vi "log analysis_gps.vi"() -> ()   [LabVIEW 2018] (continued)
02000000,471d,15824;INS_ALIGNMENT_COMPLETE,INS_RTKFIXED,37.37068991155,126.72418127348,10.1440,22.3000,0.1660,-0.2361,-0.0346,-1.526557069,-2.043657004,301.319503447,0.4414,0.2936,0.5516,0.1147,0.0924,0.0773,0.0985,0.1037,4.8734,0f000001,0*5a4270f2\n\tsystem status\tnormal 2 28.000000 0 0\trobot status\t296.398114\t62.114495\t10.144000\t-1.526557\t-2.043657\t148.680497\t0.295000\t0.017000\n\t\n15:32:29.0\tlog_raw\tgps_raw\t\tsystem status\tnormal 2 28.000000 0 0\trobot status\t296.298636\t62.188359\t10.138000\t-1.401985\t-1.954148\t148.698075\t0.220000\t0.059000\n\t\n15:32:29.5\tlog_raw\tgps_raw\t\tsystem status\tnormal 2 28.000000 0 0\trobot status\t296.178072\t62.274593\t10.135400\t-1.361112\t-1.441905\t148.768068\t0.319000\t-0.040000\n\t\n15:32:30.0\tlog_raw\tgps_raw\t\tsystem status\tnormal 2 28.000000 0 0\trobot status\t296.075944\t62.352617\t10.130400\t-0.894382\t-1.568528\t148.753681\t0.263000\t0.005000\n\t\n15:32:30.5\tlog_raw\tgps_raw\t\tsystem status\tnormal 2 28.000000 0 0\trobot status\t295.964048\t62.434825\t10.132000\t-0.800917\t-1.256471\t148.752232\t0.304000\t-0.008000\n\t\n15:32:31.0\tlog_raw\tgps_raw\t\tsystem status\tnormal 2 28.000000 0 0\trobot status\t295.846178\t62.519865\t10.128900\t-0.939613\t-0.476224\t148.649480\t0.325000\t-0.046000\n\t\n15:32:31.5\tlog_raw\tgps_raw\t#INSPVAXA,USB3,0,52.5,FINESTEERING,2107,282769.500,02000000,471d,15824;INS_ALIGNMENT_COMPLETE,INS_RTKFIXED,37.37069431364,126.72417373673,10.1300,22.3000,0.1603,-0.2654,-0.0095,-1.268871738,-0.382060792,301.325978301,0.4464,0.2940,0.5510,0.1165,0.0927,0.0772,0.0984,0.1035,4.8643,0f000001,0*c8529f83\n\tsystem status\tnormal 2 28.000000 0 0\trobot status\t295.730521\t62.603083\t10.130000\t-1.268872\t-0.382061\t148.674022\t0.301000\t0.004000\n\t\n15:32:32.0\tlog_raw\tgps_raw\t\tsystem status\tnormal 2 28.000000 0 0\trobot status\t295.610868\t62.688092\t10.129000\t-1.384299\t-0.069981\t148.517098\t0.277000\t0.034000\n\t\n15:32:32.5\tlog_raw\tgps_raw\t\tsystem status\tnormal 2 28.000000 0 0\trobot status\t295.511357\t62.766081\t10.129700\t-1.066903\t0.012632\t148.592458\t0.294000\t-0.014000\n\t\n15:32:33.0\tlog_raw\tgps_raw\t\tsystem status\tnormal 2 28.000000 0 0\trobot status\t295.383113\t62.858245\t10.131300\t-1.221038\t-0.290292\t148.364562\t0.294000\t0.000000\n\t\n15:32:33.5\tlog_raw\tgps_raw\t#INSPVAXA,USB3,0,50.5,FINESTEERING,2107,282771.500,02000000,471d,15824;INS_ALIGNMENT_COMPLETE,INS_RTKFIXED,37.37069745960,126.72416836041,10.1313,22.3000,0.1734,-0.2561,-0.0200,-1.398091128,-0.585991174,301.767912429,0.4476,0.2943,0.5503,0.1154,0.0929,0.0772,0.0983,0.1033,4.8370,0f000001,0*46dd6173\n\tsystem status\tnormal 2 28.000000 0 0\trobot status\t295.254296\t62.952253\t10.131300\t-1.398091\t-0.585991\t148.232088\t0.306000\t0.007000\n\t\n15:32:34.0\tlog_raw\tgps_raw\t\tsystem status\tnormal 2 28.000000 0 0\trobot status\t295.144963\t63.032491\t10.131200\t-1.462857\t-0.836220\t148.096342\t0.289000\t-0.005000\n\t\n15:32:34.5\tlog_raw\tgps_raw\t\tsystem status\tnormal 2 28.000000 0 0\trobot status\t295.028200\t63.124039\t10.132500\t-1.207624\t-0.963061\t148.048115\t0.304000\t-0.003000\n\t\n15:32:35.0\tlog_raw\tgps_raw\t\tsystem status\tnormal 2 28.000000 0 0\trobot status\t294.908639\t63.216920\t10.132200\t-1.135657\t-1.024801\t147.963073\t0.305000\t0.001000\n\t\n15:32:35.5\tlog_raw\tgps_raw\t\tsystem status\tnormal 2 28.000000 0 0\trobot status\t294.793362\t63.307918\t10.132000\t-0.998560\t-1.105906\t147.899852\t0.305000\t0.003000\n\t\n15:32:36.0\tlog_raw\tgps_raw\t#INSPVAXA,USB3,0,48.0,FINESTEERING,2107,282774.000,02000000,471d,15824;INS_ALIGNMENT_COMPLETE,INS_RTKFIXED,37.37070158360,126.72416168804,10.1302,22.3000,0.1865,-0.2187,-0.0076,-0.878281232,-1.102464115,302.124757826,0.4458,0.2946,0.5497,0.1138,0.0924,0.0771,0.0982,0.1032,4.8072,0f000001,0*778beed4\n\tsystem status\tnormal 2 28.000000 0 0\trobot status\t294.663268\t63.409974\t10.130200\t-0.878281\t-1.102464\t147.875242\t0.297000\t0.008000\n\t\n15:32:36.5\tlog_raw\tgps_raw\t#INSPVAXA,USB3,0,51.0,FINESTEERING,2107,282774.500,02000000,471d,15824;INS_ALIGNMENT_COMPLETE,INS_RTKFIXED,37.37070240562,126.72416038344,10.1301,22.3000,0.1841,-0.2216,-0.0074,-0.755916604,-1.039971548,302.079440422,0.4445,0.2942,0.5497,0.1137,0.0923,0.0771,0.0982,0.1032,4.7994,0f000001,0*7d8abcba\n\tsystem status\tnormal 2 28.000000 0 0\trobot status\t294.547709\t63.501210\t10.130100\t-0.755917\t-1.039972\t147.920560\t0.257000\t0.069000\n\t\n15:32:37.0\tlog_raw\tgps_raw\t\tsystem status\tnormal 2 28.000000 0 0\trobot status\t294.441010\t63.584632\t10.130300\t-0.657644\t-1.098371\t147.886694\t0.256000\t0.071000\n\t\n15:32:37.5\tlog_raw\tgps_raw\t\tsystem status\tnormal 2 28.000000 0 0\trobot status\t294.326507\t63.674259\t10.129500\t-0.698609\t-0.924125\t147.966729\t0.306000\t0.009000\n\t\n15:32:38.0\tlog_raw\tgps_raw\t\tsystem status\tnormal 2 28.000000 0 0\trobot status\t294.207903\t63.767336\t10.127700\t-0.622193\t-0.914822\t148.095651\t0.389000\t-0.119000\n\t\n15:32:38.5\tlog_raw\tgps_raw\t\tsystem status\tnormal 2 28.000000 0 0\trobot status\t294.089085\t63.861289\t10.125200\t-0.528009\t-1.070164\t148.237491\t0.311000\t0.003000\n\t\n15:32:39.0\tlog_raw\tgps_raw\t#INSPVAXA,USB3,0,52.0,FINESTEERING,2107,282777.000,02000000,471d,15824;INS_ALIGNMENT_COMPLETE,INS_RTKFIXED,37.37070657070,126.72415376285,10.1217,22.3000,0.2035,-0.2369,-0.0150,-0.446978250,-1.366804369,301.502448560,0.4425,0.2939,0.5496,0.1135,0.0924,0.0771,0.0982,0.1032,4.7938,0f000001,0*25f2a73f\n\tsystem status\tnormal 2 27.900000 0 0\trobot status\t293.961268\t63.963490\t10.121700\t-0.446978\t-1.366804\t148.497551\t0.249000\t0.102000\n\t\n15:32:39.5\tlog_raw\tgps_raw\t#INSPVAXA,USB3,0,51.5,FINESTEERING,2107,282777.500,02000000,471d,15824;INS_ALIGNMENT_COMPLETE,INS_RTKFIXED,37.37070737696,126.72415245019,10.1203,22.3000,0.1993,-0.2523,-0.0201,-0.489054474,-1.485846051,301.354572444,0.4412,0.2937,0.5492,0.1134,0.0927,0.0771,0.0982,0.1032,4.7938,0f000001,0*c63e4195\n\tsystem status\tnormal 2 27.900000 0 0\trobot status\t293.844995\t64.052977\t10.120300\t-0.489054\t-1.485846\t148.645428\t0.261000\t0.068000\n\t\n15:32:40.0\tlog_raw\tgps_raw\t#INSPVAXA,USB3,0,51.5,FINESTEERING,2107,282778.000,02000000,471d,15824;INS_ALIGNMENT_COMPLETE,INS_RTKFIXED,37.37070818895,126.72415111526,10.1183,22.3000,0.1970,-0.2381,-0.0048,-0.588842364,-1.719100289,301.162178179,0.4412,0.2937,0.5492,0.1134,0.0927,0.0771,0.0982,0.1032,4.7938,0f000001,0*cff0a9c3\n\tsystem status\tnormal 2 27.900000 0 0\trobot status\t293.726749\t64.143099\t10.118300\t-0.588842\t-1.719100\t148.837822\t0.260000\t0.055000\n\t\n15:32:40.5\tlog_raw\tgps_raw\t\tsystem status\tnormal 2 27.900000 0 0\trobot status\t293.621224\t64.222231\t10.114600\t-0.699985\t-1.731559\t149.030117\t0.234000\t0.109000\n\t\n15:32:41.0\tlog_raw\tgps_raw\t\tsystem status\tnormal 2 27.900000 0 0\trobot status\t293.505904\t64.308514\t10.110100\t-0.736273\t-1.630904\t149.356604\t0.241000\t0.105000\n\t\n15:32:41.5\tlog_raw\tgps_raw\t\tsystem status\tnormal 2 27.900000 0 0\trobot status\t293.392001\t64.394601\t10.106100\t-0.697006\t-1.585321\t149.593266\t0.253000\t0.078000\n\t\n15:32:42.0\tlog_raw\tgps_raw\t#INSPVAXA,USB3,0,45.0,FINESTEERING,2107,282780.000,02000000,471d,15824;INS_ALIGNMENT_COMPLETE,INS_RTKFIXED,37.37071131338,126.72414591828,10.1018,22.3000,0.1785,-0.2324,-0.0069,-0.645891836,-1.424803808,300.174839081,0.4413,0.2936,0.5502,0.1138,0.0926,0.0771,0.0982,0.1032,4.7947,0f000001,0*1d8f369d\n\tsystem status\tnormal 2 27.900000 0 0\trobot status\t293.266409\t64.489879\t10.101800\t-0.645892\t-1.424804\t149.825161\t0.271000\t0.042000\n\t\n15:32:42.5\tlog_raw\tgps_raw\t#INSPVAXA,USB3,0,47.0,FINESTEERING,2107,282780.500,02000000,471d,15824;INS_ALIGNMENT_COMPLETE,INS_RTKFIXED,37.37071208302,126.72414463488,10.0975,22.3000,0.1821,-0.2419,-0.0019,-0.556153794,-1.244614265,299.928543824,0.4419,0.2936,0.5508,0.1139,0.0925,0.0772,0.0982,0.1033,4.7946,0f000001,0*8f6fb982\n\tsystem status\tnormal 2 27.900000 0 0\trobot status\t293.152727\t64.575301\t10.097500\t-0.556154\t-1.244614\t150.071456\t0.269000\t0.063000\n\t\n15:32:43.0\tlog_raw\tgps_raw\t\tsystem status\tnormal 2 27.900000 0 0\trobot status\t293.049344\t64.652245\t10.092300\t-0.644835\t-1.201618\t150.236627\t0.241000\t0.104000\n\t\n15:32:43.5\tlog_raw\tgps_raw\t\tsystem status\tnormal 2 27.900000 0 0\trobot status\t292.934873\t64.737506\t10.087900\t-0.697254\t-1.176763\t150.373079\t0.274000\t0.036000\n\t\n15:32:44.0\tlog_raw\tgps_raw\t\tsystem status\tnormal 2 28.000000 0 0\trobot status\t292.821781\t64.822770\t10.082600\t-0.786091\t-1.232027\t150.520228\t0.272000\t0.043000\n\t\n15:32:44.5\tlog_raw\tgps_raw\t\tsystem status\tnormal 2 28.000000 0 0\trobot status\t292.705956\t64.906619\t10.078200\t-0.895000\t-1.549317\t150.670841\t0.281000\t0.039000\n\t\n15:32:45.0\tlog_raw\tgps_raw\t\tsystem status\tnormal 2 28.000000 0 0\trobot status\t292.590094\t64.991528\t10.072700\t-1.014159\t-1.880712\t150.764788\t0.241000\t0.093000\n\t\n15:32:45.5\tlog_raw\tgps_raw\t#INSPVAXA,USB3,0,52.5,FINESTEERING,2107,282783.500,02000000,471d,15824;INS_ALIGNMENT_COMPLETE,INS_RTKFIXED,37.37071667102,126.72413686312,10.0669,22.3000,0.1872,-0.2243,-0.0265,-0.901347734,-1.882595886,299.189069382,0.4437,0.2938,0.5525,0.1145,0.0924,0.0772,0.0982,0.1033,4.7951,0f000001,0*f21a15f8\n\tsystem status\tnormal 2 27.900000 0 0\trobot status\t292.464317\t65.084523\t10.066900\t-0.901348\t-1.882596\t150.810931\t0.334000\t-0.050000\n\t\n15:32:46.0\tlog_raw\tgps_raw\t#INSPVAXA,USB3,0,52.5,FINESTEERING,2107,282784.000,02000000,471d,15824;INS_ALIGNMENT_COMPLETE,INS_RTKFIXED,37.37071744310,126.72413557177,10.0615,22.3000,0.1842,-0.2203,-0.0202,-0.879207865,-1.728416069,299.181717490,0.4437,0.2938,0.5525,0.1145,0.0924,0.0772,0.0982,0.1033,4.7951,0f000001,0*6c7250dc\n\tsystem status\tnormal 2 28.000000 0 0\trobot status\t292.349932\t65.170216\t10.061500\t-0.879208\t-1.728416\t150.818283\t0.349000\t-0.068000\n\t\n15:32:46.5\tlog_raw\tgps_raw\t\tsystem status\tnormal 2 28.000000 0 0\trobot status\t292.247312\t65.245763\t10.056700\t-0.854639\t-1.542951\t150.875128\t0.263000\t0.061000\n\t\n15:32:47.0\tlog_raw\tgps_raw\t\tsystem status\tnormal 2 28.000000 0 0\trobot status\t292.131081\t65.329733\t10.048500\t-1.142793\t-1.256443\t150.916580\t0.255000\t0.070000\n\t\n15:32:47.5\tlog_raw\tgps_raw\t\tsystem status\tnormal 2 28.000000 0 0\trobot status\t292.014685\t65.414370\t10.039300\t-1.007102\t-1.150012\t150.972707\t0.245000\t0.079000\n\t\n15:32:48.0\tlog_raw\tgps_raw\t#INSPVAXA,USB3,0,48.5,FINESTEERING,2107,282786.000,02000000,471d,15824;INS_ALIGNMENT_COMPLETE,INS_RTKFIXED,37.37072048781,126.72413033534,10.0312,22.3000,0.2068,-0.2374,-0.0322,-0.835692120,-1.272043539,298.989138355,0.4439,0.2941,0.5534,0.1141,0.0925,0.0773,0.0982,0.1033,4.7952,0f000001,0*6862fbb7\n\tsystem status\tnormal 2 28.000000 0 0\trobot status\t291.886097\t65.508148\t10.031200\t-0.835692\t-1.272044\t151.010862\t0.396000\t-0.131000\n\t\n15:32:48.5\tlog_raw\tgps_raw\t#INSPVAXA,USB3,0,50.0,FINESTEERING,2107,282786.500,02000000,471d,15824;INS_ALIGNMENT_COMPLETE,INS_RTKFIXED,37.37072125488,126.72412899591,10.0263,22.3000,0.1993,-0.2318,-0.0321,-0.677738340,-1.537504569,298.882185903,0.4440,0.2942,0.5536,0.1140,0.0923,0.0773,0.0982,0.1033,4.7960,0f000001,0*3cb3310e\n\tsystem status\tnormal 2 28.000000 0 0\trobot status\t291.767453\t65.593285\t10.026300\t-0.677738\t-1.537505\t151.117814\t0.286000\t0.021000\n\t\n15:32:49.0\tlog_raw\tgps_raw\t#INSPVAXA,USB3,0,50.0,FINESTEERING,2107,282787.000,02000000,471d,15824;INS_ALIGNMENT_COMPLETE,INS_RTKFIXED,37.37072202374,126.72412763229,10.0205,22.3000,0.2013,-0.2217,-0.0210,-0.794961813,-1.788062217,298.885711292,0.4440,0.2942,0.5536,0.1140,0.0923,0.0773,0.0982,0.1033,4.7960,0f000001,0*1f81862e\n\tsystem status\tnormal 2 28.000000 0 0\trobot status\t291.646666\t65.678621\t10.020500\t-0.794962\t-1.788062\t151.114289\t0.254000\t0.061000\n\t\n15:32:49.5\tlog_raw\tgps_raw\t#INSPVAXA,USB3,0,44.0,FINESTEERING,2107,282787.500,02000000,471d,15824;INS_ALIGNMENT_COMPLETE,INS_RTKFIXED,37.37072277220,126.72412626224,10.0147,22.3000,0.2002,-0.2137,-0.0290,-0.849980745,-1.812919554,298.887708696,0.4445,0.2943,0.5539,0.1141,0.0924,0.0773,0.0982,0.1034,4.7971,0f000001,0*c9e15001\n\tsystem status\tnormal 2 28.000000 0 0\trobot status\t291.525309\t65.761693\t10.014700\t-0.849981\t-1.812920\t151.112291\t0.307000\t-0.016000\n\t\n15:32:50.0\tlog_raw\tgps_raw\t#INSPVAXA,USB3,0,44.0,FINESTEERING,2107,282788.000,02000000,471d,15824;INS_ALIGNMENT_COMPLETE,INS_RTKFIXED,37.37072352565,126.72412491087,10.0076,22.3000,0.2060,-0.2242,-0.0325,-0.865126530,-1.802719391,298.872730955,0.4445,0.2943,0.5539,0.1141,0.0924,0.0773,0.0982,0.1034,4.7971,0f000001,0*c2266642\n\tsystem status\tnormal 2 28.000000 0 0\trobot status\t291.405607\t65.845318\t10.007600\t-0.865127\t-1.802719\t151.127269\t0.283000\t0.031000\n\t\n15:32:50.5\tlog_raw\tgps_raw\t#INSPVAXA,USB3,0,49.0,FINESTEERING,2107,282788.500,02000000,471d,15824;INS_ALIGNMENT_COMPLETE,INS_RTKFIXED,37.37072428040,126.72412354813,10.0007,22.3000,0.2098,-0.2286,-0.0305,-0.732817876,-1.872220332,298.881417220,0.4449,0.2943,0.5542,0.1142,0.0924,0.0773,0.0982,0.1034,4.7982,0f000001,0*a1e1a8aa\n\tsystem status\tnormal 2 28.000000 0 0\trobot status\t291.284897\t65.929088\t10.000700\t-0.732818\t-1.872220\t151.118583\t0.285000\t0.019000\n\t\n15:32:51.0\tlog_raw\tgps_raw\t#INSPVAXA,USB3,0,49.0,FINESTEERING,2107,282789.000,02000000,471d,15824;INS_ALIGNMENT_COMPLETE,INS_RTKFIXED,37.37072504347,126.72412218219,9.9929,22.3000,0.1951,-0.2277,-0.0250,-0.679984989,-2.019858796,298.956218881,0.4449,0.2943,0.5542,0.1142,0.0924,0.0773,0.0982,0.1034,4.7982,0f000001,0*d14e3525\n\tsystem status\tnormal 2 28.000000 0 0\trobot status\t291.163905\t66.013781\t9.992900\t-0.679985\t-2.019859\t151.043781\t0.288000\t0.011000\n\t\n15:32:51.5\tlog_raw\tgps_raw\t#INSPVAXA,USB3,0,50.5,FINESTEERING,2107,282789.500,02000000,471d,15824;INS_ALIGNMENT_COMPLETE,INS_RTKFIXED,37.37072577695,126.72412082127,9.9869,22.3000,0.2017,-0.2348,-0.0299,-0.707518535,-2.196709608,298.969096628,0.4457,0.2945,0.5546,0.1143,0.0924,0.0773,0.0982,0.1035,4.7994,0f000001,0*e2b500de\n\tsystem status\tnormal 2 28.000000 0 0\trobot status\t291.043357\t66.095190\t9.986900\t-0.707519\t-2.196710\t151.030903\t0.364000\t-0.092000\n\t\n15:32:52.0\tlog_raw\tgps_raw\t#INSPVAXA,USB3,0,50.5,FINESTEERING,2107,282790.000,02000000,471d,15824;INS_ALIGNMENT_COMPLETE,INS_RTKFIXED,37.37072651838,126.72411947234,9.9801,22.3000,0.2152,-0.2350,-0.0246,-0.689288795,-2.210478200,298.973213622,0.4457,0.2945,0.5546,0.1143,0.0924,0.0773,0.0982,0.1035,4.7994,0f000001,0*67dd8a4d\n\tsystem status\tnormal 2 28.000000 0 0\trobot status\t290.923871\t66.177482\t9.980100\t-0.689289\t-2.210478\t151.026786\t0.291000\t0.031000\n\t\n15:32:52.5\tlog_raw\tgps_raw\t#INSPVAXA,USB3,0,50.0,FINESTEERING,2107,282790.500,02000000,471d,15824;INS_ALIGNMENT_COMPLETE,INS_RTKFIXED,37.37072725997,126.72411813576,9.9737,22.3000,0.1949,-0.2238,-0.0215,-0.636862822,-2.266623064,299.084984877,0.4461,0.2946,0.5548,0.1144,0.0925,0.0773,0.0983,0.1035,4.8006,0f000001,0*d9aa8359\n\tsystem status\tnormal 2 28.000000 0 0\trobot status\t290.805479\t66.259791\t9.973700\t-0.636863\t-2.266623\t150.915015\t0.279000\t0.016000\n\t\n15:32:53.0\tlog_raw\tgps_raw\t#DUALANTENNAHEADINGA,USB3,0,50.0,FINESTEERING,2107,282791.000,02000000,d426,15824;INSUFFICIENT_OBS,NONE,-1.000000000,0.000000000,0.000000000,0.0,0.000000000,0.000000000,\"631T\",14,2,2,2,04,00,20,00*cf3d8ad9\n\tsystem status\tnormal 2 28.000000 0 0\trobot status\t290.685466\t66.345484\t9.967200\t-0.458696\t-2.242861\t150.871926\t0.285000\t0.011000\n\t\n15:32:53.5\tlog_raw\tgps_raw\t#INSPVAXA,USB3,0,49.0,FINESTEERING,2107,282791.500,02000000,471d,15824;INS_ALIGNMENT_COMPLETE,INS_RTKFIXED,37.37072877959,126.72411543719,9.9612,22.3000,0.2083,-0.2487,-0.0306,-0.425657916,-2.232797757,299.196171617,0.4458,0.2943,0.5547,0.1143,0.0925,0.0773,0.0983,0.1035,4.8018,0f000001,0*f23e3c59\n\tsystem status\tnormal 2 28.000000 0 0\trobot status\t290.566444\t66.428454\t9.961200\t-0.425658\t-2.232798\t150.803828\t0.365000\t-0.096000\n\t\n15:32:54.0\tlog_raw\tgps_raw\t#INSPVAXA,USB3,0,49.0,FINESTEERING,2107,282792.000,02000000,471d,15824;INS_ALIGNMENT_COMPLETE,INS_RTKFIXED,37.37072953138,126.72411411925,9.9544,22.3000,0.1984,-0.2313,-0.0308,-0.400223692,-2.232054336,299.272403656,0.4458,0.2943,0.5547,0.1143,0.0925,0.0773,0.0983,0.1035,4.8018,0f000001,0*da40ff02\n\tsystem status\tnormal 2 28.000000 0 0\trobot status\t290.449703\t66.511895\t9.954400\t-0.400224\t-2.232054\t150.727596\t0.324000\t-0.055000\n\t\n15:32:54.5\tlog_raw\tgps_raw\t#INSPVAXA,USB3,0,50.0,FINESTEERING,2107,282792.500,02000000,471d,15824;INS_ALIGNMENT_COMPLETE,INS_RTKFIXED,37.37073031281,126.72411271384,9.9474,22.3000,0.1838,-0.2244,-0.0278,-0.319663676,-2.204085935,299.407243986,0.4460,0.2943,0.5548,0.1143,0.0925,0.0773,0.0983,0.1036,4.8027,0f000001,0*a7b7d02c\n\tsystem status\tnormal 2 28.000000 0 0\trobot status\t290.325214\t66.598626\t9.947400\t-0.319664\t-2.204086\t150.592756\t0.282000\t0.016000\n\t\n15:32:55.0\tlog_raw\tgps_raw\t#INSPVAXA,USB3,0,50.0,FINESTEERING,2107,282793.000,02000000,471d,15824;INS_ALIGNMENT_COMPLETE,INS_RTKFIXED,37.37073105512,126.72411141845,9.9418,22.3000,0.2101,-0.2661,-0.0283,-0.304105156,-2.230574791,299.428124027,0.4460,0.2943,0.5548,0.1143,0.0925,0.0773,0.0983,0.1036,4.8027,0f000001,0*32017f41\n\tsystem status\tnormal 2 28.000000 0 0\trobot status\t290.210470\t66.681015\t9.941800\t-0.304105\t-2.230575\t150.571876\t0.321000\t-0.013000\n\t\n15:32:55.5\tlog_raw\tgps_raw\t#INSPVAXA,USB3,0,48.5,FINESTEERING,2107,282793.500,02000000,471d,15824;INS_ALIGNMENT_COMPLETE,INS_RTKFIXED,37.37073179967,126.72411009506,9.9373,22.3000,0.1839,-0.2284,-0.0293,-0.261169015,-2.357198246,299.469051976,0.4470,0.2945,0.5553,0.1144,0.0927,0.0774,0.0983,0.1036,4.8035,0f000001,0*5198649b\n\tsystem status\tnormal 2 28.000000 0 0\trobot status\t290.093247\t66.763652\t9.937300\t-0.261169\t-2.357198\t150.530948\t0.334000\t-0.072000\n\t\n15:32:56.0\tlog_raw\tgps_raw\t#INSPVAXA,USB3,0,48.5,FINESTEERING,2107,282794.000,02000000,471d,15824;INS_ALIGNMENT_COMPLETE,INS_RTKFIXED,37.37073258034,126.72410870830,9.9322,22.3000,0.1804,-0.2290,-0.0311,-0.237665421,-2.328772316,299.577236299,0.4470,0.2945,0.5553,0.1144,0.0927,0.0774,0.0983,0.1036,4.8035,0f000001,0*00fdb5a8\n\tsystem status\tnormal 2 28.000000 0 0\trobot status\t289.970410\t66.850299\t9.932200\t-0.237665\t-2.328772\t150.422764\t0.248000\t0.075000\n\t\n15:32:56.5\tlog_raw\tgps_raw\t#INSPVAXA,USB3,0,50.0,FINESTEERING,2107,282794.500,02000000,471d,15824;INS_ALIGNMENT_COMPLETE,INS_RTKFIXED,37.37073330075,126.72410740472,9.9287,22.3000,0.1893,-0.2427,-0.0278,-0.202786531,-2.243456476,299.635927133,0.4467,0.2943,0.5552,0.1145,0.0925,0.0773,0.0983,0.1036,4.8037,0f000001,0*5cb0ba92\n\tsystem status\tnormal 2 28.000000 0 0\trobot status\t289.854941\t66.930258\t9.928700\t-0.202787\t-2.243456\t150.364073\t0.259000\t0.071000\n\t\n15:32:57.0\tlog_raw\tgps_raw\t#INSPVAXA,USB3,0,50.0,FINESTEERING,2107,282795.000,02000000,471d,15824;INS_ALIGNMENT_COMPLETE,INS_RTKFIXED,37.37073403278,126.72410609803,9.9257,22.3000,0.2016,-0.2553,-0.0322,-0.209242337,-1.998269327,299.675209205,0.4467,0.2943,0.5552,0.1145,0.0925,0.0773,0.0983,0.1036,4.8037,0f000001,0*b5d55d6c\n\tsystem status\tnormal 2 28.000000 0 0\trobot status\t289.739196\t67.011506\t9.925700\t-0.209242\t-1.998269\t150.324791\t0.366000\t-0.092000\n\t\n15:32:57.5\tlog_raw\tgps_raw\t#INSPVAXA,USB3,0,47.5,FINESTEERING,2107,282795.500,02000000,471d,15824;INS_ALIGNMENT_COMPLETE,INS_RTKFIXED,37.37073477439,126.72410478765,9.9228,22.3000,0.1988,-0.2433,-0.0255,-0.169516872,-1.839910246,299.717118650,0.4468,0.2942,0.5552,0.1144,0.0925,0.0773,0.0984,0.1036,4.8041,0f000001,0*ac4c0833\n\tsystem status\tnormal 2 28.000000 0 0\trobot status\t289.623125\t67.093817\t9.922800\t-0.169517\t-1.839910\t150.282881\t0.294000\t0.009000\n\t\n15:32:58.0\tlog_raw\tgps_raw\t#DUALANTENNAHEADINGA,USB3,0,47.5,FINESTEERING,2107,282796.000,02000000,d426,15824;INSUFFICIENT_OBS,NONE,-1.000000000,0.000000000,0.000000000,0.0,0.000000000,0.000000000,\"631T\",16,2,2,2,04,00,20,00*03fa76b0\n\tsystem status\tnormal 2 28.000000 0 0\trobot status\t289.506115\t67.178459\t9.919000\t-0.086706\t-1.778248\t150.199106\t0.344000\t-0.077000\n\t\n15:32:58.5\tlog_raw\tgps_raw\t#INSPVAXA,USB3,0,49.5,FINESTEERING,2107,282796.500,02000000,471d,15824;INS_ALIGNMENT_COMPLETE,INS_RTKFIXED,37.37073628296,126.72410213089,9.9158,22.3000,0.1865,-0.2481,-0.0343,-0.084207342,-1.811662938,299.819471466,0.4465,0.2941,0.5548,0.1145,0.0924,0.0773,0.0984,0.1036,4.8046,0f000001,0*5f5dfc2c\n\tsystem status\tnormal 2 28.000000 0 0\trobot status\t289.387793\t67.261253\t9.915800\t-0.084207\t-1.811663\t150.180529\t0.279000\t0.023000\n\t\n15:32:59.0\tlog_raw\tgps_raw\t#DUALANTENNAHEADINGA,USB3,0,49.5,FINESTEERING,2107,282797.000,02000000,d426,15824;INSUFFICIENT_OBS,NONE,-1.000000000,0.000000000,0.000000000,0.0,0.000000000,0.000000000,\"631T\",11,2,2,2,04,00,20,00*3233b119\n\tsystem status\tnormal 2 28.000000 0 0\trobot status\t289.269440\t67.343968\t9.913200\t-0.205740\t-1.946328\t150.206963\t0.297000\t0.013000\n\t\n15:32:59.5\tlog_raw\tgps_raw\t#INSPVAXA,USB3,0,51.0,FINESTEERING,2107,282797.500,02000000,471d,15824;INS_ALIGNMENT_COMPLETE,INS_RTKFIXED,37.37073777614,126.72409945855,9.9099,22.3000,0.1844,-0.2371,-0.0242,-0.262384878,-2.080175298,299.815880388,0.4468,0.2941,0.5547,0.1144,0.0924,0.0773,0.0984,0.1036,4.8050,0f000001,0*8c5fb6f4\n\tsystem status\tnormal 2 28.000000 0 0\trobot status\t289.151082\t67.426981\t9.909900\t-0.262385\t-2.080175\t150.184120\t0.351000\t-0.081000\n\t\n15:33:00.0\tlog_raw\tgps_raw\t#DUALANTENNAHEADINGA,USB3,0,51.0,FINESTEERING,2107,282798.000,02000000,d426,15824;INSUFFICIENT_OBS,NONE,-1.000000000,0.000000000,0.000000000,0.0,0.000000000,0.000000000,\"631T\",13,2,2,2,04,00,20,00*54bdf9a5\n\tsystem status\tnormal 2 28.000000 0 0\trobot status\t289.032956\t67.511715\t9.906500\t-0.164979\t-2.080670\t150.180258\t0.289000\t0.011000\n\t\n15:33:00.5\tlog_raw\tgps_raw\t#DUALANTENNAHEADINGA,USB3,0,48.5,FINESTEERING,2107,282798.500,02000000,d426,15824;INSUFFICIENT_OBS,NONE,-1.000000000,0.000000000,0.000000000,0.0,0.000000000,0.000000000,\"631T\",13,2,2,2,04,00,20,00*f78b4211\n\tsystem status\tnormal 2 28.000000 0 0\trobot status\t288.916496\t67.593249\t9.904500\t-0.163734\t-2.024921\t150.175268\t0.361000\t-0.099000\n\t\n15:33:01.0\tlog_raw\tgps_raw\t#INSPVAXA,USB3,0,48.5,FINESTEERING,2107,282799.000,02000000,471d,15824;INS_ALIGNMENT_COMPLETE,INS_RTKFIXED,37.37074001096,126.72409550695,9.9018,22.3000,0.1871,-0.2390,-0.0286,-0.222837018,-2.091989069,299.851600763,0.4467,0.2941,0.5546,0.1145,0.0924,0.0773,0.0984,0.1036,4.8055,0f000001,0*154119ed\n\tsystem status\tnormal 2 28.000000 0 0\trobot status\t288.801056\t67.675024\t9.901800\t-0.222837\t-2.091989\t150.148399\t0.255000\t0.056000\n\t\n15:33:01.5\tlog_raw\tgps_raw\t#INSPVAXA,USB3,0,48.0,FINESTEERING,2107,282799.500,02000000,471d,15824;INS_ALIGNMENT_COMPLETE,INS_RTKFIXED,37.37074075005,126.72409418540,9.8978,22.3000,0.1813,-0.2293,-0.0193,-0.296668492,-2.062854317,299.895574277,0.4469,0.2941,0.5547,0.1144,0.0924,0.0773,0.0985,0.1036,4.8059,0f000001,0*557f2fd1\n\tsystem status\tnormal 2 28.000000 0 0\trobot status\t288.683995\t67.757056\t9.897800\t-0.296668\t-2.062854\t150.104426\t0.361000\t-0.110000\n\t\n15:33:02.0\tlog_raw\tgps_raw\t#INSPVAXA,USB3,0,48.0,FINESTEERING,2107,282800.000,02000000,471d,15824;INS_ALIGNMENT_COMPLETE,INS_RTKFIXED,37.37074149494,126.72409286106,9.8944,22.3000,0.1833,-0.2479,-0.0244,-0.375636327,-2.245041894,299.896302450,0.4469,0.2941,0.5547,0.1144,0.0924,0.0773,0.0985,0.1036,4.8059,0f000001,0*618fc424\n\tsystem status\tnormal 2 28.000000 0 0\trobot status\t288.566687\t67.839731\t9.894400\t-0.375636\t-2.245042\t150.103698\t0.367000\t-0.102000\n\t\n15:33:02.5\tlog_raw\tgps_raw\t#INSPVAXA,USB3,0,50.5,FINESTEERING,2107,282800.500,02000000,471d,15824;INS_ALIGNMENT_COMPLETE,INS_RTKFIXED,37.37074223493,126.72409154227,9.8930,22.3000,0.1953,-0.2548,-0.0229,-0.359173553,-2.315682427,299.885169095,0.4472,0.2942,0.5548,0.1143,0.0924,0.0774,0.0985,0.1036,4.8064,0f000001,0*7582bc0e\n\tsystem status\tnormal 2 28.000000 0 0\trobot status\t288.449871\t67.921863\t9.893000\t-0.359174\t-2.315682\t150.114831\t0.385000\t-0.113000\n\t\n15:33:03.0\tlog_raw\tgps_raw\t#INSPVAXA,USB3,0,50.5,FINESTEERING,2107,282801.000,02000000,471d,15824;INS_ALIGNMENT_COMPLETE,INS_RTKFIXED,37.37074297365,126.72409022766,9.8906,22.3000,0.1848,-0.2408,-0.0220,-0.434084237,-2.273111027,299.921855092,0.4472,0.2942,0.5548,0.1143,0.0924,0.0774,0.0985,0.1036,4.8064,0f000001,0*0e2f8a3b\n\tsystem status\tnormal 2 28.000000 0 0\trobot status\t288.333425\t68.003853\t9.890600\t-0.434084\t-2.273111\t150.078145\t0.242000\t0.082000\n\t\n15:33:03.5\tlog_raw\tgps_raw\t#INSPVAXA,USB3,0,50.5,FINESTEERING,2107,282801.500,02000000,471d,15824;INS_ALIGNMENT_COMPLETE,INS_RTKFIXED,37.37074369952,126.72408891611,9.8878,22.3000,0.1813,-0.2385,-0.0170,-0.522003899,-2.179263420,299.918840889,0.4467,0.2943,0.5547,0.1143,0.0924,0.0773,0.0985,0.1036,4.8071,0f000001,0*ee077a21\n\tsystem status\tnormal 2 28.000000 0 0\trobot status\t288.217250\t68.084418\t9.887800\t-0.522004\t-2.179263\t150.081159\t0.293000\t0.004000\n\t\n15:33:04.0\tlog_raw\tgps_raw\t#DUALANTENNAHEADINGA,USB3,0,50.5,FINESTEERING,2107,282802.000,02000000,d426,15824;INSUFFICIENT_OBS,NONE,-1.000000000,0.000000000,0.000000000,0.0,0.000000000,0.000000000,\"631T\",12,2,2,2,04,00,20,00*74fbc462\n\tsystem status\tnormal 2 28.000000 0 0\trobot status\t288.101332\t68.165999\t9.883800\t-0.536050\t-2.179465\t150.066801\t0.298000\t0.012000\n\t\n15:33:04.5\tlog_raw\tgps_raw\t#INSPVAXA,USB3,0,47.0,FINESTEERING,2107,282802.500,02000000,471d,15824;INS_ALIGNMENT_COMPLETE,INS_RTKFIXED,37.37074515687,126.72408631213,9.8800,22.3000,0.1804,-0.2401,-0.0128,-0.478381012,-2.174780645,299.958693295,0.4464,0.2943,0.5545,0.1143,0.0924,0.0773,0.0985,0.1036,4.8081,0f000001,0*e501e358\n\tsystem status\tnormal 2 28.000000 0 0\trobot status\t287.986594\t68.246169\t9.880000\t-0.478381\t-2.174781\t150.041307\t0.370000\t-0.105000\n\t\n15:33:05.0\tlog_raw\tgps_raw\t#DUALANTENNAHEADINGA,USB3,0,47.0,FINESTEERING,2107,282803.000,02000000,d426,15824;INSUFFICIENT_OBS,NONE,-1.000000000,0.000000000,0.000000000,0.0,0.000000000,0.000000000,\"631T\",13,2,2,2,04,00,20,00*accba235\n\tsystem status\tnormal 2 28.000000 0 0\trobot status\t287.870862\t68.327272\t9.875900\t-0.499817\t-2.093079\t150.035960\t0.279000\t0.026000\n\t\n15:33:05.5\tlog_raw\tgps_raw\t#DUALANTENNAHEADINGA,USB3,0,45.0,FINESTEERING,2107,282803.500,02000000,d426,15824;INSUFFICIENT_OBS,NONE,-1.000000000,0.000000000,0.000000000,0.0,0.000000000,0.000000000,\"631T\",13,2,2,2,04,00,20,00*b3511e24\n\tsystem status\tnormal 2 28.000000 0 0\trobot status\t287.755357\t68.407514\t9.873000\t-0.580082\t-2.196230\t150.036980\t0.298000\t0.000000\n\t\n15:33:06.0\tlog_raw\tgps_raw\t#INSPVAXA,USB3,0,45.0,FINESTEERING,2107,282804.000,02000000,471d,15824;INS_ALIGNMENT_COMPLETE,INS_RTKFIXED,37.37074734035,126.72408240044,9.8696,22.3000,0.1782,-0.2385,-0.0140,-0.685361203,-2.151633306,299.976720233,0.4460,0.2942,0.5542,0.1144,0.0925,0.0773,0.0985,0.1036,4.8092,0f000001,0*10ad259a\n\tsystem status\tnormal 2 28.000000 0 0\trobot status\t287.640102\t68.488513\t9.869600\t-0.685361\t-2.151633\t150.023280\t0.303000\t0.008000\n\t\n15:33:06.5\tlog_raw\tgps_raw\t#DUALANTENNAHEADINGA,USB3,0,46.0,FINESTEERING,2107,282804.500,02000000,d426,15824;INSUFFICIENT_OBS,NONE,-1.000000000,0.000000000,0.000000000,0.0,0.000000000,0.000000000,\"631T\",15,2,2,2,04,00,20,00*58397695\n\tsystem status\tnormal 2 28.000000 0 0\trobot status\t287.527787\t68.569047\t9.868100\t-0.679232\t-2.050136\t150.013013\t0.289000\t0.023000\n\t\n15:33:07.0\tlog_raw\tgps_raw\t#DUALANTENNAHEADINGA,USB3,0,46.0,FINESTEERING,2107,282805.000,02000000,d426,15824;INSUFFICIENT_OBS,NONE,-1.000000000,0.000000000,0.000000000,0.0,0.000000000,0.000000000,\"631T\",15,2,2,2,04,00,20,00*e2f26315\n\tsystem status\tnormal 2 28.000000 0 0\trobot status\t287.413455\t68.652100\t9.866600\t-0.702808\t-1.949775\t149.980106\t0.251000\t0.074000\n\t\n15:33:07.5\tlog_raw\tgps_raw\t#DUALANTENNAHEADINGA,USB3,0,44.5,FINESTEERING,2107,282805.500,02000000,d426,15824;INSUFFICIENT_OBS,NONE,-1.000000000,0.000000000,0.000000000,0.0,0.000000000,0.000000000,\"631T\",15,2,2,2,04,00,20,00*a81239c8\n\tsystem status\tnormal 2 28.000000 0 0\trobot status\t287.298608\t68.734681\t9.865200\t-0.700717\t-1.929163\t149.972736\t0.302000\t0.009000\n\t\n15:33:08.0\tlog_raw\tgps_raw\t#DUALANTENNAHEADINGA,USB3,0,44.5,FINESTEERING,2107,282806.000,02000000,d426,15824;INSUFFICIENT_OBS,NONE,-1.000000000,0.000000000,0.000000000,0.0,0.000000000,0.000000000,\"631T\",15,2,2,2,04,00,20,00*c96925fa\n\tsystem status\tnormal 2 28.000000 0 0\trobot status\t287.185294\t68.817421\t9.863300\t-0.701483\t-1.875706\t149.927856\t0.383000\t-0.110000\n\t\n15:33:08.5\tlog_raw\tgps_raw\t#INSPVAXA,USB3,0,47.5,FINESTEERING,2107,282806.500,02008000,471d,15824;INS_ALIGNMENT_COMPLETE,INS_RTKFIXED,37.37075103198,126.72407599150,9.8611,22.3000,0.1775,-0.2152,-0.0113,-0.726876844,-1.853734910,300.056532649,0.4475,0.2946,0.5549,0.1145,0.0926,0.0774,0.0984,0.1036,4.8109,0f000001,0*336afd29\n\tsystem status\tnormal 2 28.000000 0 0\trobot status\t287.072409\t68.898247\t9.861100\t-0.726877\t-1.853735\t149.943467\t0.250000\t0.070000\n\t\n15:33:09.0\tlog_raw\tgps_raw\t#DUALANTENNAHEADINGA,USB3,0,47.5,FINESTEERING,2107,282807.000,02008000,d426,15824;INSUFFICIENT_OBS,NONE,-1.000000000,0.000000000,0.000000000,0.0,0.000000000,0.000000000,\"631T\",15,2,2,2,04,00,20,00*1eefde6e\n\tsystem status\tnormal 2 28.000000 0 0\trobot status\t286.957092\t68.981374\t9.858500\t-0.779789\t-2.086978\t149.915137\t0.253000\t0.058000\n\t\n15:33:09.5\tlog_raw\tgps_raw\t#DUALANTENNAHEADINGA,USB3,0,50.5,FINESTEERING,2107,282807.500,02008000,d426,15824;INSUFFICIENT_OBS,NONE,-1.000000000,0.000000000,0.000000000,0.0,0.000000000,0.000000000,\"631T\",15,2,2,2,04,00,20,00*fe8ccb2d\n\tsystem status\tnormal 2 28.000000 0 0\trobot status\t286.841071\t69.062813\t9.856500\t-0.888203\t-2.021026\t149.885505\t0.246000\t0.071000\n\t\n15:33:10.0\tlog_raw\tgps_raw\t#INSPVAXA,USB3,0,50.5,FINESTEERING,2107,282808.000,02008000,471d,15824;INS_ALIGNMENT_COMPLETE,INS_RTKFIXED,37.37075325131,126.72407209622,9.8541,22.3000,0.1789,-0.2215,-0.0236,-0.924752960,-1.991766220,300.099829298,0.4478,0.2946,0.5550,0.1144,0.0926,0.0774,0.0984,0.1036,4.8105,0f000001,0*94ebbe09\n\tsystem status\tnormal 2 28.000000 0 0\trobot status\t286.727372\t69.144570\t9.854100\t-0.924753\t-1.991766\t149.900171\t0.259000\t0.055000\n\t\n15:33:10.5\tlog_raw\tgps_raw\t#DUALANTENNAHEADINGA,USB3,0,50.0,FINESTEERING,2107,282808.500,02008000,d426,15824;INSUFFICIENT_OBS,NONE,-1.000000000,0.000000000,0.000000000,0.0,0.000000000,0.000000000,\"631T\",14,2,2,2,04,00,20,00*7e4f9fbd\n\tsystem status\tnormal 2 28.000000 0 0\trobot status\t286.613572\t69.225605\t9.851400\t-0.967220\t-1.935302\t149.889513\t0.391000\t-0.155000\n\t\n15:33:11.0\tlog_raw\tgps_raw\t#DUALANTENNAHEADINGA,USB3,0,50.0,FINESTEERING,2107,282809.000,02008000,d426,15824;INSUFFICIENT_OBS,NONE,-1.000000000,0.000000000,0.000000000,0.0,0.000000000,0.000000000,\"631T\",14,2,2,2,04,00,20,00*c4848a3d\n\tsystem status\tnormal 2 28.000000 0 0\trobot status\t286.496891\t69.309534\t9.847500\t-0.931690\t-1.832535\t149.868639\t0.415000\t-0.177000\n\t\n15:33:11.5\tlog_raw\tgps_raw\t#DUALANTENNAHEADINGA,USB3,0,48.0,FINESTEERING,2107,282809.500,02008000,d426,15824;INSUFFICIENT_OBS,NONE,-1.000000000,0.000000000,0.000000000,0.0,0.000000000,0.000000000,\"631T\",14,2,2,2,04,00,20,00*568c01e1\n\tsystem status\tnormal 2 28.000000 0 0\trobot status\t286.382614\t69.391548\t9.844700\t-0.872134\t-1.807390\t149.847977\t0.270000\t0.040000\n\t\n15:33:12.0\tlog_raw\tgps_raw\t#DUALANTENNAHEADINGA,USB3,0,48.0,FINESTEERING,2107,282810.000,02008000,d426,15824;INSUFFICIENT_OBS,NONE,-1.000000000,0.000000000,0.000000000,0.0,0.000000000,0.000000000,\"631T\",14,2,2,2,04,00,20,00*cb078c5f\n\tsystem status\tnormal 2 28.000000 0 0\trobot status\t286.269475\t69.473317\t9.842400\t-0.947006\t-1.839613\t149.841963\t0.390000\t-0.144000\n\t\n15:33:12.5\tlog_raw\tgps_raw\t#INSPVAXA,USB3,0,50.0,FINESTEERING,2107,282810.500,02008000,471d,15824;INS_ALIGNMENT_COMPLETE,INS_RTKFIXED,37.37075697026,126.72406559815,9.8397,22.3000,0.1784,-0.2281,-0.0276,-0.963357433,-2.013990950,300.156490692,0.4474,0.2946,0.5550,0.1144,0.0925,0.0774,0.0983,0.1035,4.8086,0f000001,0*76b7c623\n\tsystem status\tnormal 2 28.000000 0 0\trobot status\t286.151783\t69.557336\t9.839700\t-0.963357\t-2.013991\t149.843509\t0.318000\t-0.064000\n\t\n15:33:13.0\tlog_raw\tgps_raw\t#DUALANTENNAHEADINGA,USB3,0,50.0,FINESTEERING,2107,282811.000,02008000,d426,15824;INSUFFICIENT_OBS,NONE,-1.000000000,0.000000000,0.000000000,0.0,0.000000000,0.000000000,\"631T\",14,2,2,2,04,00,20,00*e3c41203\n\tsystem status\tnormal 2 28.000000 0 0\trobot status\t286.034269\t69.641399\t9.836900\t-1.088886\t-2.023235\t149.839861\t0.295000\t0.002000\n\t\n15:33:13.5\tlog_raw\tgps_raw\t#DUALANTENNAHEADINGA,USB3,0,50.0,FINESTEERING,2107,282811.500,02008000,d426,15824;INSUFFICIENT_OBS,NONE,-1.000000000,0.000000000,0.000000000,0.0,0.000000000,0.000000000,\"631T\",15,2,2,2,04,00,20,00*e3358302\n\tsystem status\tnormal 2 28.000000 0 0\trobot status\t285.918179\t69.724857\t9.833700\t-0.962975\t-2.045756\t149.859684\t0.253000\t0.068000\n\t\n15:33:14.0\tlog_raw\tgps_raw\t#DUALANTENNAHEADINGA,USB3,0,50.0,FINESTEERING,2107,282812.000,02008000,d426,15824;INSUFFICIENT_OBS,NONE,-1.000000000,0.000000000,0.000000000,0.0,0.000000000,0.000000000,\"631T\",15,2,2,2,04,00,20,00*824e9f30\n\tsystem status\tnormal 2 28.000000 0 0\trobot status\t285.803528\t69.807588\t9.829600\t-0.889335\t-2.011789\t149.904196\t0.334000\t-0.060000\n\t\n15:33:14.5\tlog_raw\tgps_raw\t#DUALANTENNAHEADINGA,USB3,0,50.0,FINESTEERING,2107,282812.500,02008000,d426,15824;INSUFFICIENT_OBS,NONE,-1.000000000,0.000000000,0.000000000,0.0,0.000000000,0.000000000,\"631T\",14,2,2,2,04,00,20,00*82bf0e31\n\tsystem status\tnormal 2 27.900000 0 0\trobot status\t285.685624\t69.891836\t9.825200\t-0.745478\t-1.940124\t149.938204\t0.421000\t-0.178000\n\t\n15:33:15.0\tlog_raw\tgps_raw\t#DUALANTENNAHEADINGA,USB3,0,50.0,FINESTEERING,2107,282813.000,02008000,d426,15824;INSUFFICIENT_OBS,NONE,-1.000000000,0.000000000,0.000000000,0.0,0.000000000,0.000000000,\"631T\",12,2,2,2,04,00,20,00*a5a810a2\n\tsystem status\tnormal 2 28.000000 0 0\trobot status\t285.569063\t69.974938\t9.819800\t-0.814872\t-1.930768\t149.941273\t0.410000\t-0.166000\n\t\n15:33:15.5\tlog_raw\tgps_raw\t#DUALANTENNAHEADINGA,USB3,0,48.0,FINESTEERING,2107,282813.500,02008000,d426,15824;INSUFFICIENT_OBS,NONE,-1.000000000,0.000000000,0.000000000,0.0,0.000000000,0.000000000,\"631T\",11,2,2,2,04,00,20,00*94f61dd7\n\tsystem status\tnormal 2 28.000000 0 0\trobot status\t285.451484\t70.056599\t9.814700\t-0.866674\t-1.940719\t149.938238\t0.201000\t0.138000\n\t\n15:33:16.0\tlog_raw\tgps_raw\t#INSPVAXA,USB3,0,48.0,FINESTEERING,2107,282814.000,02008000,471d,15824;INS_ALIGNMENT_COMPLETE,INS_RTKFIXED,37.37076222900,126.72405635034,9.8094,22.3000,0.1883,-0.2144,-0.0181,-0.772460660,-2.046540094,300.011288466,0.4470,0.2944,0.5548,0.1144,0.0924,0.0774,0.0982,0.1035,4.8080,0f000001,0*4e4fcada\n\tsystem status\tnormal 2 28.000000 0 0\trobot status\t285.332627\t70.141003\t9.809400\t-0.772461\t-2.046540\t149.988712\t0.328000\t-0.051000\n\t\n15:33:16.5\tlog_raw\tgps_raw\t#INSPVAXA,USB3,0,50.0,FINESTEERING,2107,282814.500,02000000,471d,15824;INS_ALIGNMENT_COMPLETE,INS_RTKFIXED,37.37076300208,126.72405500228,9.8062,22.3000,0.1859,-0.2191,-0.0086,-0.683595212,-2.119791281,300.037756065,0.4472,0.2945,0.5552,0.1144,0.0924,0.0774,0.0982,0.1035,4.8084,0f000001,0*aac7df20\n\tsystem status\tnormal 2 28.000000 0 0\trobot status\t285.213218\t70.226807\t9.806200\t-0.683595\t-2.119791\t149.962244\t0.372000\t-0.110000\n\t\n15:33:17.0\tlog_raw\tgps_raw\t#DUALANTENNAHEADINGA,USB3,0,50.0,FINESTEERING,2107,282815.000,02000000,d426,15824;INSUFFICIENT_OBS,NONE,-1.000000000,0.000000000,0.000000000,0.0,0.000000000,0.000000000,\"631T\",13,2,2,2,04,00,20,00*d37808cc\n\tsystem status\tnormal 2 28.000000 0 0\trobot status\t285.096694\t70.312174\t9.802700\t-0.595570\t-2.177562\t149.959768\t0.286000\t0.026000\n\t\n15:33:17.5\tlog_raw\tgps_raw\t#DUALANTENNAHEADINGA,USB3,0,49.0,FINESTEERING,2107,282815.500,02000000,d426,15824;INSUFFICIENT_OBS,NONE,-1.000000000,0.000000000,0.000000000,0.0,0.000000000,0.000000000,\"631T\",12,2,2,2,04,00,20,00*f2d6d5ec\n\tsystem status\tnormal 2 28.000000 0 0\trobot status\t284.979385\t70.395845\t9.798900\t-0.578455\t-2.160583\t150.003542\t0.283000\t0.028000\n\t\n15:33:18.0\tlog_raw\tgps_raw\t#DUALANTENNAHEADINGA,USB3,0,49.0,FINESTEERING,2107,282816.000,02000000,d426,15824;INSUFFICIENT_OBS,NONE,-1.000000000,0.000000000,0.000000000,0.0,0.000000000,0.000000000,\"631T\",13,2,2,2,04,00,20,00*444f4986\n\tsystem status\tnormal 2 28.000000 0 0\trobot status\t284.860675\t70.480739\t9.793700\t-0.632938\t-2.162391\t149.978897\t0.291000\t0.020000\n\t\n15:33:18.5\tlog_raw\tgps_raw\t#DUALANTENNAHEADINGA,USB3,0,52.0,FINESTEERING,2107,282816.500,02000000,d426,15824;INSUFFICIENT_OBS,NONE,-1.000000000,0.000000000,0.000000000,0.0,0.000000000,0.000000000,\"631T\",12,2,2,2,04,00,20,00*ad6839ee\n\tsystem status\tnormal 2 28.000000 0 0\trobot status\t284.744203\t70.564207\t9.790000\t-0.568209\t-2.043363\t149.974717\t0.374000\t-0.103000\n\t\n15:33:19.0\tlog_raw\tgps_raw\t#DUALANTENNAHEADINGA,USB3,0,52.0,FINESTEERING,2107,282817.000,02000000,d426,15824;INSUFFICIENT_OBS,NONE,-1.000000000,0.000000000,0.000000000,0.0,0.000000000,0.000000000,\"631T\",14,2,2,2,04,00,20,00*8a7f277d\n\tsystem status\tnormal 2 28.000000 0 0\trobot status\t284.629630\t70.648349\t9.785400\t-0.442570\t-2.134504\t150.007168\t0.326000\t-0.038000\n\t\n15:33:19.5\tlog_raw\tgps_raw\t#DUALANTENNAHEADINGA,USB3,0,47.0,FINESTEERING,2107,282817.500,02000000,d426,15824;INSUFFICIENT_OBS,NONE,-1.000000000,0.000000000,0.000000000,0.0,0.000000000,0.000000000,\"631T\",13,2,2,2,04,00,20,00*e8ab143d\n\tsystem status\tnormal 2 28.000000 0 0\trobot status\t284.510021\t70.734578\t9.780300\t-0.350306\t-2.338700\t150.002612\t0.278000\t0.019000\n\t\n15:33:20.0\tlog_raw\tgps_raw\t#DUALANTENNAHEADINGA,USB3,0,47.0,FINESTEERING,2107,282818.000,02000000,d426,15824;INSUFFICIENT_OBS,NONE,-1.000000000,0.000000000,0.000000000,0.0,0.000000000,0.000000000,\"631T\",11,2,2,2,04,00,20,00*49573191\n\tsystem status\tnormal 2 28.000000 0 0\trobot status\t284.391874\t70.820058\t9.774900\t-0.395280\t-2.299498\t149.965963\t0.269000\t0.046000\n\t\n15:33:20.5\tlog_raw\tgps_raw\t#DUALANTENNAHEADINGA,USB3,0,45.5,FINESTEERING,2107,282818.500,02000000,d426,15824;INSUFFICIENT_OBS,NONE,-1.000000000,0.000000000,0.000000000,0.0,0.000000000,0.000000000,\"631T\",11,2,2,2,04,00,20,00*03b76b4c\n\tsystem status\tnormal 2 28.000000 0 0\trobot status\t284.276474\t70.904256\t9.770300\t-0.320786\t-2.351462\t149.946266\t0.376000\t-0.115000\n\t\n15:33:21.0\tlog_raw\tgps_raw\t#DUALANTENNAHEADINGA,USB3,0,45.5,FINESTEERING,2107,282819.000,02000000,d426,15824;INSUFFICIENT_OBS,NONE,-1.000000000,0.000000000,0.000000000,0.0,0.000000000,0.000000000,\"631T\",12,2,2,2,04,00,20,00*1a2af865\n\tsystem status\tnormal 2 28.000000 0 0\trobot status\t284.160387\t70.988968\t9.764800\t-0.332761\t-2.313351\t149.959057\t0.283000\t0.014000\n\t\n15:33:21.5\tlog_raw\tgps_raw\t#DUALANTENNAHEADINGA,USB3,0,50.5,FINESTEERING,2107,282819.500,02000000,d426,15824;INSUFFICIENT_OBS,NONE,-1.000000000,0.000000000,0.000000000,0.0,0.000000000,0.000000000,\"631T\",13,2,2,2,04,00,20,00*e522c036\n\tsystem status\tnormal 2 28.000000 0 0\trobot status\t284.041735\t71.071786\t9.758700\t-0.333060\t-2.280613\t149.974007\t0.237000\t0.079000\n\t\n15:33:22.0\tlog_raw\tgps_raw\t#DUALANTENNAHEADINGA,USB3,0,50.5,FINESTEERING,2107,282820.000,02000000,d426,15824;INSUFFICIENT_OBS,NONE,-1.000000000,0.000000000,0.000000000,0.0,0.000000000,0.000000000,\"631T\",14,2,2,2,04,00,20,00*1723a46a\n\t
